vi "Gray if False.vi"(11 "Grayed Out?":bool) -> (3 "Enabled State":T1(ring))   [LabVIEW 2020, in "VI Properties Editor.lvlib"]
doc: "Outputs either Enabled or Disabled and Grayed out based on <B>Grayed Out?</B>."
uses:
  VI Properties Editor.lvlib
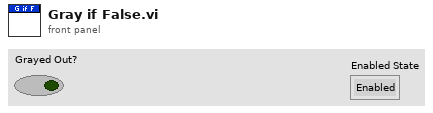
[diagram p1: front panel]
types:
  T1 = enum8{"Enabled", "Disabled", "Disabled and Grayed Out"}
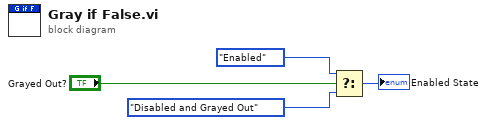
[diagram p0: block diagram]
diagram:
  n1 = Select(t=T1."Enabled" ("Disabled"), s="Grayed Out?", f=T1."Disabled and Grayed Out" ("Disabled")) -> (s? t:f=→"Enabled State":T1)
